vi "Axis_Go Point.vi"(11 "RobotPoints in":string[](array[string])) -> (0 "error out":errorcluster)   [LabVIEW 2019]
uses:
  LLB/Commonly VI/FilterPointNameToFloat.vi
panel:
  in  "error in (no error)":errorcluster
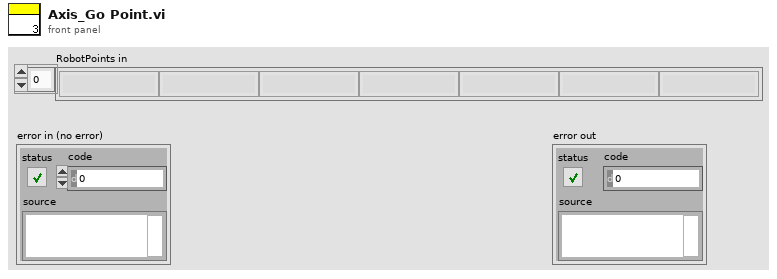
[diagram p1: front panel]
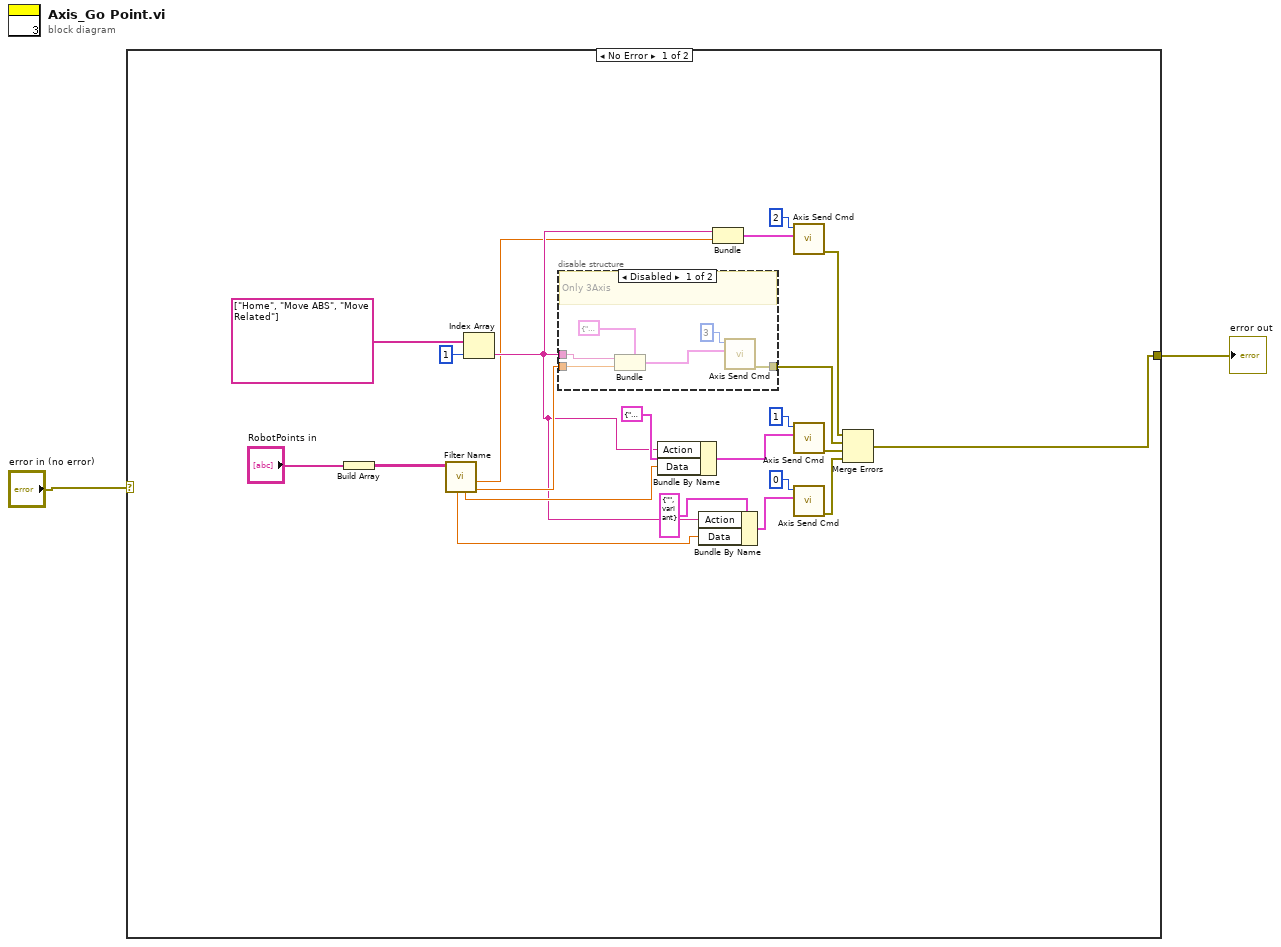
[diagram p0: block diagram]
diagram:
  n1 = case shown="No Error" "error in (no error)" {
    selector: "error in (no error)" -> [_ w31]
    tunnel: [w17 w31] -> w2
    frame No Error {
      n2 = Build Array("RobotPoints in") -> (w15:string[][])
      n3 = call-poly "Filter Name.vi"("RobotPoints in"=w15) -> ("U"=w19:dbl, "Z"=w10:dbl, "Y"=w20:dbl, "X"=w21:dbl)  [unwired: 4 in, 3 out]
      n4 = Index Array(array=string[] ["Home", "Move ABS", "Move Related"], index=1) -> (element=w11:string)
      n5 = disable-structure shown="Disabled" {
        disable-tunnel: w19 -> [w26 _]
        disable-tunnel: w11 -> [w27 _]
        disable-tunnel: [w29 _] -> w18
        frame Disabled {
          # "Only 3Axis"
          n6 = Bundle(cluster=cluster{"Action":string, "Data":variant} {"Action"="", "Data"=variant} ("element"), "Action"=w27, "Data"=w26) -> (w25:cluster{"Action":string, "Data":variant})
          n7 = call "Axis Send Cmd.vi"("DataIn"=w25, "Axis Index"=3) -> ("Error Out"=w29:errorcluster)  [unwired: 9 in]
        }
        frame Enabled {
        }
      }
      n8 = Bundle By Name(cluster=cluster{"Action":string, "Data":variant} {"Action"="", "Data"=variant} ("element"), "Action"=w11, "Data"=w20) -> (w7:cluster{"Action":string, "Data":variant})
      n9 = Bundle By Name(cluster=cluster{"Action":string, "Data":variant} {"Action"="", "Data"=variant} ("element"), "Action"=w11, "Data"=w21) -> (w4:cluster{"Action":string, "Data":variant})
      n10 = Bundle(w11, "Z"=w10) -> (w9:cluster{string, "Z":dbl})  [unwired: 1 in]
      n11 = call "Axis Send Cmd.vi"("DataIn"=w9, "Axis Index"=2) -> ("Error Out"=w13:errorcluster)  [unwired: 9 in]
      n12 = call "Axis Send Cmd.vi"("DataIn"=w7, "Axis Index"=1) -> ("Error Out"=w6:errorcluster)  [unwired: 9 in]
      n13 = call "Axis Send Cmd.vi"("DataIn"=w4, "Axis Index"=0) -> ("Error Out"=w3:errorcluster)  [unwired: 9 in]
      n14 = Merge Errors(w13, w18, w6, w3) -> (w17:errorcluster)
    }
    frame Error {
    }
  }
  "error out" <- w2
